vi "Dashboard Main.vi"() -> ()   [LabVIEW 2017]
uses:
  <vilib>/Utility/miscctls.llb/LVRowAndColumnTypeDef.ctl
  <vilib>/event_ctls.llb/eventvkey.ctl
  <vilib>/Rock Robotics/Network Tables/NT Read Numeric Array.vi
  <vilib>/Rock Robotics/Network Tables/NT Read Boolean Array.vi
  <vilib>/Rock Robotics/Network Tables/NT Write Boolean Array.vi
  <vilib>/Utility/file.llb/Read Delimited Spreadsheet (DBL).vi
  <vilib>/Rock Robotics/Network Tables/NT Write Numeric Array.vi
  <vilib>/Utility/file.llb/Write Delimited Spreadsheet (DBL).vi
  <vilib>/Rock Robotics/WPI/Dashboard/WPI_DashboardLogging Global.vi
panel:
  in  "Camera Settings Right":T1={"Frame Rate"=30, "Compression"=30, "Size"=1, "DB Camera Config"=FALSE} {"Frame Rate" scale=1.0..30.0; "Compression" scale=100.0..-1.0; "Size" items=["640x480", "320x240", "160x120"]}
  in  "Camera Name Right":string(combo)="No Camera Selection"
  out "Camera Info":cluster{"Mbps LED":bool, "Mbps":dbl, "fps":dbl} {"fps" format="%#.1g"; "Mbps" format="%#.1g"}
  in  "Camera Settings":T1={"Frame Rate"=30, "Compression"=30, "Size"=1, "DB Camera Config"=FALSE} {"Frame Rate" scale=1.0..30.0; "Compression" scale=100.0..-1.0; "Size" items=["640x480", "320x240", "160x120"]}
  in  "TCP":refnum<k5>
  in  "Rec Mode":enum32{"Stop", "Record", "Playback"}(radio)
  out "Robot IP":string
  out "Image Message":string="Timeout in Camera Communications"
  in  "Dashboard Tab":T2(tab)
  out "NT Connection":bool
  out "MotorChart R":cluster{"Numeric":dbl, "Numeric":dbl}(graph)
  out "MotorChart L":cluster{"Numeric":dbl, "Numeric":dbl}(graph)
  out "MotorSliders R":cluster{"MotorSlide1":dbl, "MotorSlide2":dbl} {"MotorSlide2" scale=-1.0..1.0 scale format="%#_2e"; "MotorSlide1" scale=-1.0..1.0 scale format="%#_2e"}
  out "MotorSliders L":cluster{"MotorSlide1":dbl, "MotorSlide2":dbl} {"MotorSlide2" scale=-1.0..1.0 scale format="%#_2e"; "MotorSlide1" scale=-1.0..1.0 scale format="%#_2e"}
  out "JS1 Z":dbl(slide) scale=-1.0..1.0 scale format="%#_2e"
  out "JS1 Graph":cluster{"X":dbl, "Y":dbl}[](graph)
  out "JS1 Buttons":T3
  out "JS2 Z":dbl(slide) scale=-1.0..1.0 scale format="%#_2e"
  out "JS2 Graph":cluster{"X":dbl, "Y":dbl}[](graph)
  out "JS2 Buttons":T3
  out "Mode":T4(ring)=enum."Auto Disabled"
  out "Gear State":string="Waiting...."
  out "Ramps":bool[](array[boolean])
  out "Camera Image Right":T5(plugin-control)
  in  "DB/String 9":string
  in  "DB/String 8":string
  in  "DB/String 7":string
  in  "DB/String 6":string
  in  "DB/String 5":string
  in  "DB/String 4":string
  in  "DB/String 3":string
  in  "DB/String 2":string
  in  "DB/String 1":string
  in  "DB/String 0":string
  in  "DB/Slider 0":dbl(slide) scale=0.0..5.0
  in  "DB/Slider 1":dbl(slide) scale=0.0..5.0
  in  "DB/Slider 2":dbl(slide) scale=0.0..5.0
  in  "DB/Slider 3":dbl(slide) scale=0.0..5.0
  out "DB/LED 3":bool
  out "DB/LED 2":bool
  out "DB/LED 1":bool
  out "DB/LED 0":bool
  in  "DB/Button 3":bool
  in  "DB/Button 2":bool
  in  "DB/Button 1":bool
  in  "DB/Button 0":bool caption="New Name"
  in  "Test Slider":dbl(slide) scale=0.0..100.0 scale format="%#_3g"
  in  "On/Off":bool caption="Solenoid"
  in  "Test Name":u16(ring) items=["Select the test to run..."]
  in  "Test Tree":string(tree)
  in  "Motor":cluster{"Value":dbl, "Enable":bool} {"Value" scale=-1.0..1.0 scale format="%#_3g"}
  out "Progress":T6 {"Test Progress" scale=0.0..100.0}
  in  "Rev/Fwd":cluster{"Forward":bool, "Reverse":bool}
  in  "Test Ring":u16(ring) items=["Monochrome", "Color"]
  out "Cmd Status":string
  in  "Execute Command":bool
  in  "Command Params":string[][](table)
  in  "Command Selection":i32(listbox)
  in  "CheckList":i32(listbox)
  out "Tree":string(tree)
  out "new picture":picture
  in  "Starting Pos":i16(slide)=128 scale=340.0..50.0
  in  "Right String":string
  in  "Left String":string
  in  "Load Left Auto":bool
  in  "Save Left Auto":bool
  in  "Save Right Auto":bool
  in  "Load Right Auto":bool
  in  "Select Auto":string(combo)="Select Autonomous ..."
  in  "Turn":dbl[](array[slide]) scale=0.0..1.0
  out "Speed Tuning":cluster{"yi":dbl[], "ramp data":dbl[]}[](graph)
  out "Rotation Tuning":cluster{"yi":dbl[], "ramp data":dbl[]}[](graph)
  in  "Ramps":bool
  in  "Shifting":bool
  in  "STOP":bool
  in  "Save":bool
  in  "Speed":dbl[](array[slide]) scale=0.0..1.0
  in  "Load":bool
  out "Camera Image":T5(plugin-control)
  out "Background":bool
  in  "Camera Name":string(combo)="No Camera Selection"
  # "HW"
  # "HW"
  # "Joysticks"
  # "Drive Motors"
  # "Front"
  # "Right"
  # "Left"
  # "Back"
  # "This tab is a great place for autonomous settings and robot-specific values.\nPlace controls and indicators inside this tab and match name to\nDashboard Variables on robot. You can also delete this comment."
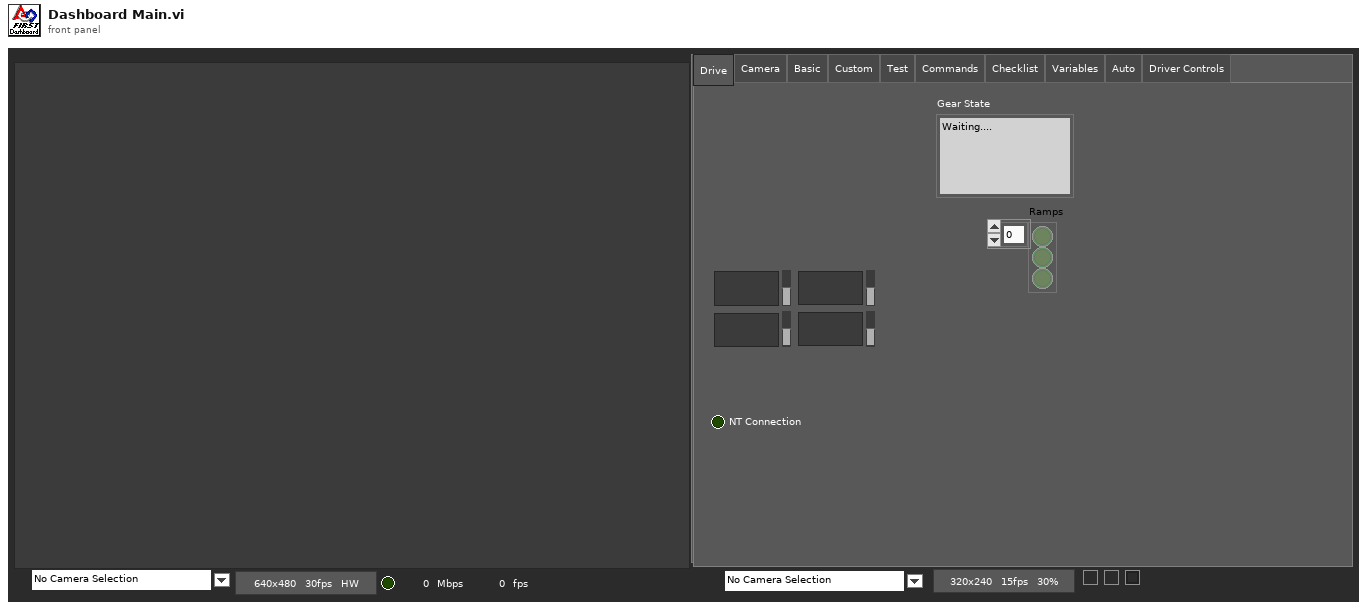
[diagram p1: front panel]
types:
  T1 = cluster{"Frame Rate":i32, "Compression":i32, "Size":u16, "DB Camera Config":bool}
  T2 = enum32{"Drive", "Camera", "Basic", "Custom", "Test", "Commands", "Checklist", "Variables", "Auto", "Driver Controls"}
  T3 = cluster{bool, bool, bool, bool, bool, bool, bool, bool, bool, bool, bool, bool}
  T4 = enum8{"Tele-Op Disabled", "Tele-Op Enabled", "Auto Disabled", "Auto Enabled", "Test Disabled", "Test Enabled", "Disconnected", "No Code", "E-Stop"}
  T5 = typedef "IMAQ Image.ctl" = refnum<image>
  T6 = cluster{"Test Progress":u8, "Test Progress Text":string}
  T7 = cluster{"Save Path":path, "Interval (s)":dbl, "Keep":i32}
  T8 = enum32{"Drive", "Camera", "Basic", "Custom", "Test", "Commands", "Checklist", "Variables"}
  T9 = typedef "Image Type" = u32
  T10 = cluster{"IDs":cluster{"RPC field ID":u16, "Unique ID":u16}, "String":string}
  T11 = cluster{"Error Strings":string, "Disable Counts":cluster{u16, u16}, "Rail Faults":cluster{u16, u16, u16}, "Robot IP":string, "DB Mode":u8, "Event Info":cluster{"Name":string, "Type":u8, "Number":u16, "Replay":u8}}
  T12 = cluster{"Storage":cluster{"Disk Free":u64, "RAM Block":u32, "RAM free":u32}, "CPU Utilization":cluster{"CPU % ISR":sgl, "CPU % Time Crit":sgl, "CPU % Timed Str":sgl, "CPU % High":sgl, "CPU % Above":sgl, "CPU % Normal":sgl, "CPU % Low":sgl}, "CAN":cluster{"% Bus Utilization":sgl, "Bus Off Cnt":u32, "TX_FIFO Full Cnt":u32, "Receive Error Cnt":u8, "Transmit Error Cnt":u8}, "HID":cluster{"HID Outputs":u32, "Rumble Low":u16, "Rumble High":u16}[]}
  T13 = cluster{"Status bits":cluster{"Test Mode":bool, "Autonomous":bool, "Enabled":bool, "Code Start":bool, "Brownout":bool, "Reserved 2":bool, "Reserved 3":bool, "E-Stop":bool}, "Code Trace":cluster{"Disabled":bool, "TeleOp":bool, "Auto":bool, "Test":bool}, "Controller Type":enum16{"unknown", "cRIO", "roboRio"}, "Code?":enum16{"unknown", "noCode", "code"}, "Battery V":dbl}
  T14 = cluster{"Control Bits":cluster{"TestMode":bool, "Autonomous":bool, "Enabled":bool, "FMS Present":bool, bool, bool, bool, "E-Stop":bool}, "Team Station ":u8, "Countdown":sgl, "Joystick Values":cluster{"Axes":dbl[], "Buttons":bool[], "POVs":i16[]}[]}
  T15 = cluster{"Axes":dbl[], "Buttons":bool[], "POVs":i16[]}[]
  T16 = cluster{"Axes":dbl[], "Buttons":bool[], "POVs":i16[]}
  T17 = cluster{"Buttons[0]":bool, "Buttons[1]":bool, "Buttons[2]":bool, "Buttons[3]":bool, "Buttons[4]":bool, "Buttons[5]":bool, "Buttons[6]":bool, "Buttons[7]":bool, "Buttons[8]":bool, "Buttons[9]":bool, "Buttons[10]":bool, "Buttons[11]":bool}
  T18 = typedef "LVBoundsTypeDef.ctl" = cluster{"Width":u32, "Height":u32}
  T19 = cluster{"Camera Image":refnum<vi>, "Dashboard Tab":refnum<vi>, "Background":refnum<vi>, "Rec Mode":refnum<vi>, "Test Slider":refnum<vi>, "On/Off ":refnum<vi>, "Test Ring":refnum<vi>, "Rev/Fwd":refnum<vi>, "Test Name":refnum<vi>, "Motor":refnum<vi>, "Progress":refnum<vi>, "CheckList":refnum<vi>, "Tree":refnum<vi>, "Test Tree":refnum<vi>, "Command Params":refnum<vi>, "Command Selection":refnum<vi>, "Execute Command":refnum<vi>, "Cmd Status":refnum<vi>, "Camera Settings":refnum<vi>, "Camera Name":refnum<vi>, "Camera Info":refnum<vi>, "Camera Settings Right":refnum<vi>, "Camera Name Right":refnum<vi>, "Camera Image Right":refnum<vi>}
  T20 = cluster{"Camera Name":string, string, "Saved DB Images Info":cluster{"Save Path":path, "Interval (s)":dbl, "Keep":i32}}
  T21 = cluster{"Camera Name Right":string, string, "Saved DB Images Info":cluster{"Save Path":path, "Interval (s)":dbl, "Keep":i32}}
  T22 = cluster{"Operation":enum16{"Update", "Clear"}, "Color Box":u32}[]
  T23 = typedef "eventvkey.ctl" = enum16{"ASCII", "Enter", "Return", "Shift", "Ctrl", "Alt", "Cmd", "Opt", "Caps", "NumLock", "Clear", "Break", "Up", "Down", "Left", "Right", "Insert", "Delete", "Home", "End", "PageUp", "PageDown", "Escape", "Help", "Pause", "ScrollLock", "F1", "F2", "F3", "F4", "F5", "F6", "F7", "F8", "F9", "F10", "F11", "F12", "F13", "F14", "F15", "F16", "F17", "F18", "F19", "F20", "F21", "F22", "F23", "F24", "Play", "VolumeUp", "VolumeDown", "Mute", "Two Byte Char"}
  T24 = cluster{"Image Size":bool, "Image Type":bool, "Pixel Value":bool, "ROI Information":bool, "Zoom Factor":bool}
  T25 = cluster{"Operation":enum16{"Update", "Clear"}, "Color Box":u32}
  T26 = typedef "LVRowAndColumnTypeDef.ctl" = cluster{"Row":i32, "Column":i32}
  T27 = cluster{"Shift":bool, "Ctrl":bool, "Alt":bool, "Cmd":bool, "Opt":bool}
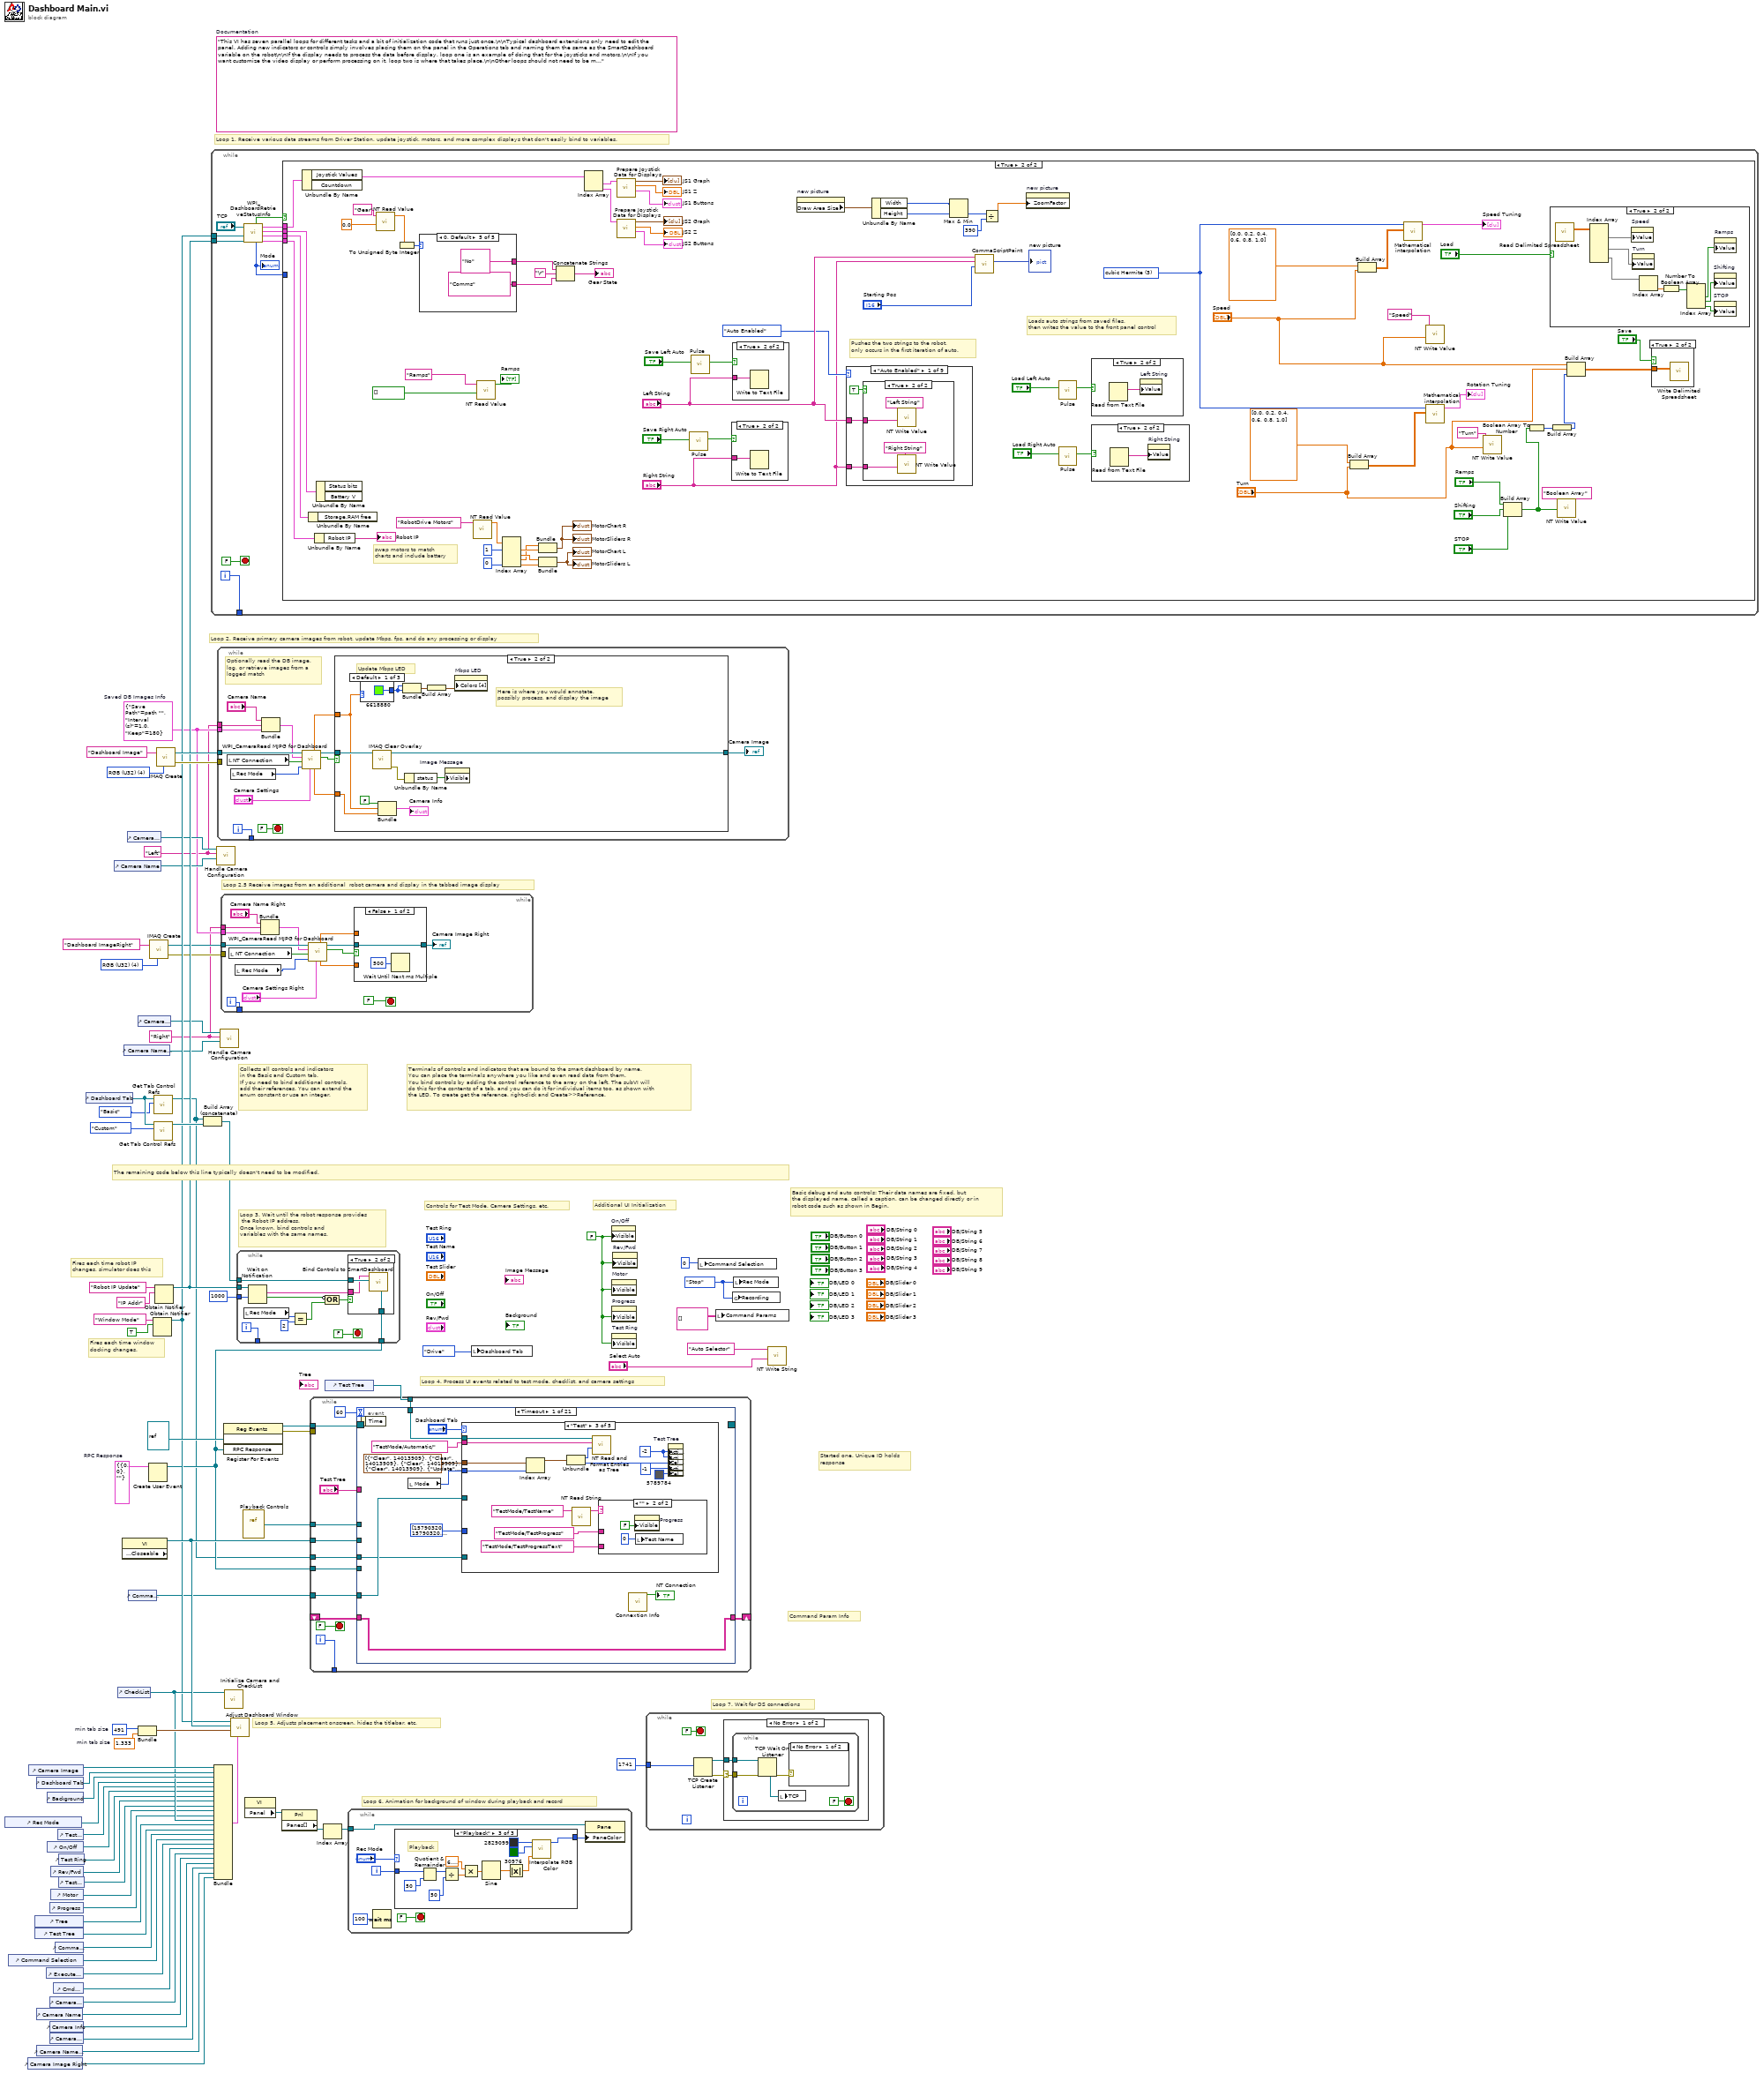
[diagram p0: block diagram]
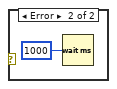
[diagram p3: hidden frame]
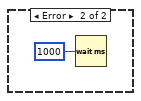
[diagram p4: hidden frame]
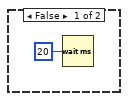
[diagram p5: hidden frame]
diagram:
  w3 = T7 {"Save Path"=path "", "Interval (s)"=1.0, "Keep"=180}  # Saved DB Images Info
  w2 = "Right"
  w1 = "Left"
  w13 = T9 4 items=["Grayscale (U8)", "Grayscale (I16)", "Grayscale (SGL)", "Complex (CSG)", "RGB (U32)", "HSL (U32)", "RGB (U64)"] ("Image Type")
  w29 = T10 {"IDs"={"RPC field ID"=0, "Unique ID"=0}, "String"=""}  # RPC Response
  w52 = 491  # min tab size
  w51 = 1.333  # min tab size
  w59 = enum32{"Stop", "Record", "Playback"}."Stop" ("Rec Mode")
  w36 = FALSE ("Visible")
  (unwired) "This VI has seven parallel loops for different tasks and a bit of initialization code that runs just once.\n\nTypical dashboard extensions only need to edit the panel. Adding new indicators or controls simply involves placing them on the panel in the Operations tab and naming them the same as the SmartDashboard variable on the robot\n\nIf the display needs to process the data before display, loop one is an example of doing that for the joysticks and motors.\n\nIf you want customize the video display or perform processing on it, loop two is where that takes place.\n\nOther loops should not need to be modified. They are pretty standard, and document the task they perform."  # Documentation
  w76 = T9 4 items=["Grayscale (U8)", "Grayscale (I16)", "Grayscale (SGL)", "Complex (CSG)", "RGB (U32)", "HSL (U32)", "RGB (U64)"] ("Image Type")
  # "Loop 2.5 Receive images from an additional  robot camera and display in the tabbed image display"
  # "Command Param Info"
  # "Started one, Unique ID holds\nresponse"
  # "Loop 7. Wait for DS connections"
  # "Basic debug and auto controls: Their data names are fixed, but\nthe displayed name, called a caption, can be changed directly or in\nrobot code such as shown in Begin."
  # "Controls for Test Mode, Camera Settings, etc."
  # "Additional UI Initialization"
  # "Loop 6. Animation for background of window during playback and record"
  # "Fires each time robot IP\nchanges, simulator does this"
  # "Fires each time window\ndocking changes."
  # "Collects all controls and indicators\nin the Basic and Custom tab.\nIf you need to bind additional controls,\nadd their references. You can extend the\nenum constant or use an integer."
  # "The remaining code below this line typically doesn't need to be modified."
  # "Loop 4. Process UI events related to test mode, checklist, and camera settings"
  # "Terminals of controls and indicators that are bound to the smart dashboard by name.\nYou can place the terminals anywhere you like and even read data from them.\nYou bind controls by adding the control reference to the array on the left. The subVI will\ndo this for the contents of a tab, and you can do it for individual items too, as shown with\nthe LED. To create get the reference, right-click and Create>>Reference."
  # "Loop 3. Wait until the robot response provides\n the Robot IP address.\nOnce known, bind controls and\nvariables with the same names."
  # "Loop 5. Adjusts placement onscreen, hides the titlebar, etc."
  # "Loop 1. Receive various data streams from Driver Station, update joystick, motors, and more complex displays that don't easily bind to variables."
  # "Loop 2. Receive primary camera images from robot, update Mbps, fps, and do any processing or display"
  n1 = control-ref of="Rec Mode"() -> (w42:refnum<vi>)
  n2 = control-ref of="Command Selection"() -> (w28:refnum<vi>)
  n3 = control-ref of="Camera Image Right"() -> (w6:refnum<vi>)
  n4 = control-ref of="Camera Image"() -> (w54:refnum<vi>)
  n5 = control-ref of="Tree"() -> (w46:refnum<vi>)
  n6 = control-ref of="Test Tree"() -> (w45:refnum<vi>)
  n7 = control-ref of="Dashboard Tab"() -> (w53:refnum<vi>)
  n8 = control-ref of="Camera Name"() -> (w19:refnum<vi>)
  n9 = control-ref of="Camera Name Right"() -> (w7:refnum<vi>)
  n10 = control-ref of="Execute Command"() -> (w30:refnum<vi>)
  n11 = control-ref of="Background"() -> (w49:refnum<vi>)
  n12 = control-ref of="On/Off"() -> (w40:refnum<vi>)
  n13 = control-ref of="Progress"() -> (w37:refnum<vi>)
  n14 = control-ref of="Camera Settings"() -> (w20:refnum<vi>)
  n15 = control-ref of="Camera Info"() -> (w18:refnum<vi>)
  n16 = control-ref of="Camera Settings Right"() -> (w8:refnum<vi>)
  n17 = control-ref of="Rev/Fwd"() -> (w38:refnum<vi>)
  n18 = control-ref of="Motor"() -> (w43:refnum<vi>)
  n19 = control-ref of="Cmd Status"() -> (w24:refnum<vi>)
  n20 = control-ref of="Command Params"() -> (w31:refnum<vi>)
  n21 = control-ref of="Test Slider"() -> (w41:refnum<vi>)
  n22 = control-ref of="Test Ring"() -> (w39:refnum<vi>)
  n23 = control-ref of="Test Name"() -> (w44:refnum<vi>)
  n24 = control-ref of="Dashboard Tab"() -> (w57:refnum<vi>)
  n25 = control-ref of="Camera Name"() -> (w21:refnum<vi>)
  n26 = control-ref of="CheckList"() -> (w47:refnum<vi>)
  n27 = property class="VI" props=["Front Panel.Closeable"]() -> (reference out=w58:refnum<vi>)  [unwired: 2 in, 2 out]
  n28 = control-ref of="Camera Name Right"() -> (w9:refnum<vi>)
  n29 = control-ref of="Camera Settings"() -> (w22:refnum<vi>)
  n30 = control-ref of="Command Params"() -> (w23:refnum<vi>)
  n31 = control-ref of="Camera Settings Right"() -> (w10:refnum<vi>)
  n32 = Bundle("min tab size"=w52, "min tab size"=w51) -> (w50:cluster{"min tab size":i32, "min tab size":dbl})  [unwired: 1 in]
  n33 = Create User Event(user event datatype=w29) -> (user event=w25:refnum<user-event>)  [unwired: 1 in, 1 out]
  n34 = call "IMAQ Create"("Image Name"="Dashboard ImageRight", "Image Type"=w13) -> ("New Image"=w12:T5, "error out"=w11:errorcluster)  [unwired: 2 in, 1 out]
  n35 = Obtain Notifier(name (unnamed)="Window Mode", notification data type=TRUE) -> (notifier out=w34:refnum<notifier>)  [unwired: 2 in, 2 out]
  n36 = call <vilib>:"Get Tab Control Refs.vi"("Page Index"=T8."Basic" ("Dashboard Tab"), "TabControl in"=w57) -> ("ControlsOnPage"=w17:refnum<vi>[])  [unwired: 9 in]
  n37 = call <vilib>:"Get Tab Control Refs.vi"("Page Index"=T8."Custom" ("Dashboard Tab"), "TabControl in"=w57) -> ("ControlsOnPage"=w56:refnum<vi>[])  [unwired: 9 in]
  n38 = Obtain Notifier(name (unnamed)="Robot IP Update", notification data type="IP Addr" ("name (unnamed)")) -> (notifier out=w35:refnum<notifier>)  [unwired: 2 in, 2 out]
  n39 = call "IMAQ Create"("Image Name"="Dashboard Image", "Image Type"=w76) -> ("New Image"=w74:T5, "error out"=w73:errorcluster)  [unwired: 2 in, 1 out]
  n40 = Build Array (concatenate)(w17, w56) -> (w55:refnum<vi>[])
  n41 = while {
    tunnel: [w86] -> _
    tunnel: w35 -> [w80]
    tunnel: w34 -> [w77]
    i -> [w86]
    stop <- FALSE stop-if-true
    n42 = call <vilib>:"WPI_DashboardRetrieveStatusInfo.vi"("Binding Refnum"=w80, "Window Mode Notifier"=w77, "TCP Cnx"="TCP") -> ("Power and Errors"=w81:T11, "Robot Metrics"=w84:T12, "Status Info"=w85:T13, "Control Info"=w82:T14, "Robot Mode"=w79:T4, "Process?"=w83:bool)  [unwired: 3 in]
    "Mode" <- w79
    n43 = case shown="True" w83 {
      tunnel: w85 -> [_ w163]
      tunnel: w84 -> [_ w162]
      tunnel: w82 -> [_ w161]
      tunnel: w81 -> [_ w160]
      tunnel: w79 -> [_ _]
      frame False {
        n44 = Wait (ms)(milliseconds to wait=u32 20) -> ()  [unwired: 1 out]
      }
      frame True {
        w109 = 3 items=["nearest", "linear", "spline", "cubic Hermite", "Lagrange"] ("Method")
        # "Pushes the two strings to the robot,\nonly occurs in the first iteration of auto."
        # "Loads auto strings from saved files,\nthen writes the value to the front panel control"
        # "swap motors to match\ncharts and include battery"
        n45 = Unbundle By Name(w161) -> ("Joystick Values"=w151:T15)  [unwired: 1 out]
        n46 = Unbundle By Name(w162) -> ()  [unwired: 1 out]
        n47 = Unbundle By Name(w160) -> ("Robot IP"=→"Robot IP":string)
        n48 = Unbundle By Name(w163) -> ()  [unwired: 2 out]
        n49 = call-poly <vilib>:"NT Read Value.vi"("Default Value"=0.0, "Name"="Gear") -> ("Numeric"=w138:dbl)  [unwired: 8 in, 1 out]
        n50 = To Unsigned Byte Integer(number=w138) -> (unsigned 8bit integer=w139:u8)
        n51 = case shown="0, Default" w139 {
          tunnel: ["Low" "High" "Low" "High" "No"] -> w135
          tunnel: ["Manual" "Manual" "Automatic" "Automatic" "Comms"] -> w133
          frame 1 {
          }
          frame 2 {
          }
          frame 3 {
          }
          frame 4 {
          }
          frame 0, Default {
          }
        }
        n52 = call-poly <vilib>:"NT Read Value.vi"("Name"="RobotDrive Motors") -> ("Numeric Array"=w141:dbl[])  [unwired: 9 in, 1 out]
        n53 = call-poly <vilib>:"NT Read Value.vi"("Default Value"=bool[] [], "Name"="Ramps") -> ("Boolean Array"=→"Ramps":bool[])  [unwired: 8 in, 1 out]
        n54 = Index Array(array=w141, index #1=1, index #4=0) -> (element #1=w155:dbl, element #2=w156:dbl, element #3=w154:dbl, element #4=w159:dbl)  [unwired: 2 in]
        n55 = Bundle("Numeric"=w154, "Numeric"=w155) -> (→"MotorChart R" →"MotorSliders R":cluster{"Numeric":dbl, "Numeric":dbl})  [unwired: 1 in]
        n56 = Bundle("Numeric"=w156, "Numeric"=w159) -> (→"MotorChart L" →"MotorSliders L":cluster{"Numeric":dbl, "Numeric":dbl})  [unwired: 1 in]
        n57 = Concatenate Strings(w135, "\r", w133) -> (→"Gear State":string)
        n58 = Index Array(array=w151) -> (element #1=w150:T16, element #2=w146:T16)  [unwired: 2 in]
        n59 = call "Prepare Joystick Data for Displays.vi"("Joystick Values"=w146) -> ("Buttons"=→"JS2 Buttons":T17, "Z Axis"=→"JS2 Z":dbl, "Cartesian Data"=→"JS2 Graph":cluster{"X axis":dbl, "X axis":dbl}[])  [unwired: 8 in]
        n60 = call "Prepare Joystick Data for Displays.vi"("Joystick Values"=w150) -> ("Buttons"=→"JS1 Buttons":T17, "Z Axis"=→"JS1 Z":dbl, "Cartesian Data"=→"JS1 Graph":cluster{"X axis":dbl, "X axis":dbl}[])  [unwired: 8 in]
        n61 = call "Pulse.vi"("Input"="Save Right Auto") -> ("Output"=w126:bool)  [unwired: 10 in]
        n62 = call "Pulse.vi"("Input"="Save Left Auto") -> ("Output"=w122:bool)  [unwired: 10 in]
        n63 = case shown="True" w126 {
          tunnel: "Right String" -> [_ w181]
          frame False {
          }
          frame True {
            n64 = Write to Text File(text=w181) -> ()  [unwired: 3 in, 3 out]
          }
        }
        n65 = case shown="True" w122 {
          tunnel: "Left String" -> [_ w184]
          frame False {
          }
          frame True {
            n66 = Write to Text File(text=w184) -> ()  [unwired: 3 in, 3 out]
          }
        }
        n67 = property on="new picture" class="Pict"() -> ("Draw Area Size"=w114:T18)  [unwired: 2 in, 2 out]
        n68 = case shown="\"Auto Enabled\"" T4."Auto Enabled" ("Robot Mode") {
          tunnel: "Left String" -> [w176 _ _ _ _ _ _ _ _]
          tunnel: "Right String" -> [w175 _ _ _ _ _ _ _ _]
          frame "Auto Enabled" {
            n69 = case shown="True" TRUE {
              tunnel: w176 -> [_ w180]
              tunnel: w175 -> [_ w179]
              frame False {
              }
              frame True {
                n70 = call-poly <vilib>:"NT Write Value.vi"("String"=w180, "Name"="Left String") -> ()  [unwired: 9 in, 1 out]
                n71 = call-poly <vilib>:"NT Write Value.vi"("String"=w179, "Name"="Right String") -> ()  [unwired: 9 in, 1 out]
              }
            }
          }
          frame "Test Disabled" {
          }
          frame "Test Enabled" {
          }
          frame "Disconnected" {
          }
          frame "No Code" {
          }
          frame "E-Stop" {
          }
          frame "Auto Disabled" {
          }
          frame "Tele-Op Enabled" {
          }
          frame "Tele-Op Disabled" {
          }
        }
        n72 = Unbundle By Name(w114) -> ("Width"=w118:u32, "Height"=w117:u32)
        n73 = Max & Min(x=w118, y=w117) -> (min(x,y)=w116:u32)  [unwired: 1 out]
        n74 = call "CommaScriptPaint.vi"("Starting Pos"="Starting Pos", "string 2"="Right String", "string"="Left String") -> ("new picture"=→"new picture":picture)  [unwired: 7 in, 1 out]
        n75 = Divide(x=w116, y=u32 390) -> (x/y=w113:dbl)
        n76 = property on="new picture" class="Pict"("ZoomFactor"=w113) -> ()  [unwired: 2 in, 2 out]
        n77 = call "Pulse.vi"("Input"="Load Left Auto") -> ("Output"=w123:bool)  [unwired: 10 in]
        n78 = call "Pulse.vi"("Input"="Load Right Auto") -> ("Output"=w129:bool)  [unwired: 10 in]
        n79 = case shown="True" w123 {
          frame False {
          }
          frame True {
            n80 = Read from Text File() -> (text=w183:string)  [unwired: 4 in, 3 out]
            n81 = property on="Left String" class="Str"("Value"=w183) -> ()  [unwired: 2 in, 2 out]
          }
        }
        n82 = case shown="True" w129 {
          frame False {
          }
          frame True {
            n83 = Read from Text File() -> (text=w182:string)  [unwired: 4 in, 3 out]
            n84 = property on="Right String" class="Str"("Value"=w182) -> ()  [unwired: 2 in, 2 out]
          }
        }
        n85 = Build Array(dbl[] [0.0, 0.2, 0.4, 0.6, 0.8, 1.0] ("Speed 2"), "Turn") -> (w91:dbl[][])
        n86 = Build Array(dbl[] [0.0, 0.2, 0.4, 0.6, 0.8, 1.0] ("Speed 2"), "Speed") -> (w100:dbl[][])
        n87 = call "Mathematical interpolation.vi"("Input data"=w100, "Method"=w109) -> ("1D Interpolation Graph"=→"Speed Tuning":cluster{"yi":dbl[], "ramp data":dbl[]}[])  [unwired: 8 in, 1 out]
        n88 = call-poly <vilib>:"NT Write Value.vi"("Numeric Array"="Speed", "Name"="Speed") -> ()  [unwired: 9 in, 1 out]
        n89 = call "Mathematical interpolation.vi"("Input data"=w91, "Method"=w109) -> ("1D Interpolation Graph"=→"Rotation Tuning":cluster{"yi":dbl[], "ramp data":dbl[]}[])  [unwired: 8 in, 1 out]
        n90 = call-poly <vilib>:"NT Write Value.vi"("Numeric Array"="Turn", "Name"="Turn") -> ()  [unwired: 9 in, 1 out]
        n91 = Build Array("Ramps", "Shifting", "STOP") -> (w99:bool[])
        n92 = Boolean Array To Number(Boolean array=w99) -> (number=w98:u32)
        n93 = case shown="True" "Load" {
          frame False {
          }
          frame True {
            n94 = call-poly <vilib>:"Read Delimited Spreadsheet.vi"() -> ("all rows"=w172:dbl[][])  [unwired: 10 in, 5 out]
            n95 = Index Array(array=w172) -> (element #1=w171:dbl[], element #2=w170:dbl[], element #3=w169:dbl[])  [unwired: 6 in]
            n96 = property on="Speed" class="Arr (strict)"("Value"=w171) -> ()  [unwired: 2 in, 2 out]
            n97 = property on="Turn" class="Arr (strict)"("Value"=w170) -> ()  [unwired: 2 in, 2 out]
            n98 = Index Array(array=w169) -> (element=w168:dbl)  [unwired: 1 in]
            n99 = Number To Boolean Array(number=w168) -> (Boolean array=w167:bool[])
            n100 = Index Array(array=w167) -> (element #1=w166:bool, element #2=w165:bool, element #3=w164:bool)  [unwired: 3 in]
            n101 = property on="Shifting" class="Bool (strict)"("Value"=w165) -> ()  [unwired: 2 in, 2 out]
            n102 = property on="STOP" class="Bool (strict)"("Value"=w164) -> ()  [unwired: 2 in, 2 out]
            n103 = property on="Ramps" class="Bool (strict)"("Value"=w166) -> ()  [unwired: 2 in, 2 out]
          }
        }
        n104 = Build Array(w98) -> (w97:u32[])
        n105 = call-poly <vilib>:"NT Write Value.vi"("Boolean Array"=w99, "Name"="Boolean Array") -> ()  [unwired: 9 in, 1 out]
        n106 = Build Array("Speed", "Turn", w97) -> (w96:dbl[][])
        n107 = case shown="True" "Save" {
          tunnel: w96 -> [_ w173]
          frame False {
          }
          frame True {
            n108 = call-poly <vilib>:"Write Delimited Spreadsheet.vi"("2D data"=w173) -> ()  [unwired: 13 in, 2 out]
          }
        }
      }
    }
  }
  n109 = Bundle("Camera Image"=w54, "Dashboard Tab"=w53, "Background"=w49, "Rec Mode"=w42, "Test Slider"=w41, "On/Off"=w40, "Test Ring"=w39, "Rev/Fwd"=w38, "Test Name"=w44, "Motor"=w43, "Progress"=w37, "CheckList"=w47, "Tree"=w46, "Test Tree"=w45, "Command Params"=w31, "Command Selection"=w28, "Execute Command"=w30, "Cmd Status"=w24, "Camera Settings"=w20, "Camera Name"=w19, "Camera Info"=w18, "Camera Settings Right"=w8, "Camera Name Right"=w7, "Camera Image Right"=w6) -> (w48:T19)  [unwired: 1 in]
  n110 = call "Handle Camera Configuration.vi"("CameraNameRef"=w21, "Display Name"=w1, "ClusterRef"=w22) -> ()  [unwired: 9 in]
  n111 = while {
    tunnel: w74 -> [w207]
    tunnel: w73 -> [_]
    tunnel: [w208] -> _
    tunnel: w3 -> [w198]
    tunnel: w1 -> [w195]
    i -> [w208]
    stop <- FALSE stop-if-true
    # "Optionally read the DB image,\nlog, or retrieve images from a\nlogged match"
    n112 = local read "NT Connection"() -> (w199:bool)
    n113 = local read "Rec Mode"() -> (w203:enum32{"Stop", "Record", "Playback"})
    n114 = Bundle("Camera Name"="Camera Name", w195, "Saved DB Images Info"=w198) -> (w197:T20)  [unwired: 1 in]
    n115 = call <vilib>:"WPI_CameraRead MJPG for Dashboard.vi"("Camera Settings"="Camera Settings", "Rec Mode"=w203, "NT Connection"=w199, "Capture Info"=w197, "Refnum in"=w207) -> ("Active"=w205:bool, "Refnum out"=w206:T5, "FPS"=w204:dbl, "Bandwidth (Mbps)"=w202:dbl)  [unwired: 3 in]
    n116 = case shown="True" w205 {
      tunnel: w206 -> [w210 w221]
      tunnel: w202 -> [_ w218]
      tunnel: w204 -> [_ w219]
      tunnel: [w210 w215] -> w200
      frame False {
        w212 = u32 1985280 ("Color Box")
        # "Sleep for 500ms"
        n117 = Bundle("Color Box"=w212, "Color Box"=w212) -> (w213:cluster{"Color Box":u32, "Color Box":u32})  [unwired: 1 out]
        n118 = Build Array(w213) -> (w211:cluster{"Color Box":u32, "Color Box":u32}[])
        n119 = property on="Mbps LED" class="Bool (strict)"("Colors [4]"=w211) -> ()  [unwired: 2 in, 2 out]
        n120 = Wait Until Next ms Multiple(millisecond multiple=u32 500) -> ()  [unwired: 1 out]
      }
      frame True {
        # "Here is where you would annotate,\npossibly process, and display the image"
        # "Update Mbps LED"
        n121 = case shown="Default" w218 {
          tunnel: [u32 6618880 ("Color Box") u32 16776722 ("Color Box") u32 16716800 ("Color Box")] -> w222
          frame Default {
          }
          frame 4, 5 {
          }
          frame 6.. {
          }
        }
        n122 = call "IMAQ Clear Overlay"("Image"=w221) -> ("error out"=w224:errorcluster, "Image Out"=w215:T5)  [unwired: 2 in, 7 out]
        n123 = Bundle(FALSE, "Bandwidth (Mbps)"=w218, "FPS"=w219) -> (→"Camera Info":cluster{bool, "Bandwidth (Mbps)":dbl, "FPS":dbl})  [unwired: 1 in]
        n124 = Bundle("Color Box"=w222, "Color Box"=w222) -> (w223:cluster{"Color Box":u32, "Color Box":u32})  [unwired: 1 out]
        n125 = Unbundle By Name(w224) -> ("status"=w225:bool)
        n126 = Build Array(w223) -> (w220:cluster{"Color Box":u32, "Color Box":u32}[])
        n127 = property on="Image Message" class="Str"("Visible"=w225) -> ()  [unwired: 2 in, 2 out]
        n128 = property on="Mbps LED" class="Bool (strict)"("Colors [4]"=w220) -> ()  [unwired: 2 in, 2 out]
      }
    }
    "Camera Image" <- w200
  }
  n129 = call "Handle Camera Configuration.vi"("CameraNameRef"=w9, "Display Name"=w2, "ClusterRef"=w10) -> ()  [unwired: 9 in]
  n130 = while {
    tunnel: w12 -> [w243]
    tunnel: w11 -> [_]
    tunnel: [w238] -> _
    tunnel: w3 -> [w232]
    tunnel: w2 -> [w229]
    i -> [w238]
    stop <- FALSE stop-if-true
    n131 = local read "NT Connection"() -> (w233:bool)
    n132 = local read "Rec Mode"() -> (w242:enum32{"Stop", "Record", "Playback"})
    n133 = Bundle("Camera Name Right"="Camera Name Right", w229, "Saved DB Images Info"=w232) -> (w231:T21)  [unwired: 1 in]
    n134 = call <vilib>:"WPI_CameraRead MJPG for Dashboard.vi"("Camera Settings"="Camera Settings Right", "Rec Mode"=w242, "NT Connection"=w233, "Capture Info"=w231, "Refnum in"=w243) -> ("Active"=w237:bool, "Refnum out"=w240:T5, "FPS"=w235:dbl, "Bandwidth (Mbps)"=w236:dbl)  [unwired: 3 in]
    n135 = case shown="False" w237 {
      tunnel: w240 -> [w244 w246]
      tunnel: w236 -> [_ _]
      tunnel: w235 -> [_ _]
      tunnel: [w244 w246] -> w234
      frame False {
        n136 = Wait Until Next ms Multiple(millisecond multiple=u32 500) -> ()  [unwired: 1 out]
      }
      frame True {
      }
    }
    "Camera Image Right" <- w234
  }
  n137 = register-events(refnum<vi> refnum, w25) -> (reference out=w63:refnum<event-registration>, error out=w62:errorcluster)  [unwired: 2 in]
  n138 = call "Initialize Camera and CheckList.vi"("ListBox in"=w47) -> ()  [unwired: 11 in]
  n139 = call "Adjust Dashboard Window.vi"("Sizing Refnums"=w48, "Size Constraints"=w50, "VI"=w58, "WIn Mode"=w34) -> ()  [unwired: 8 in]
  n140 = while {
    tunnel: w55 -> [w258]
    tunnel: w35 -> [w256]
    tunnel: [w254] -> _
    tunnel: u32 1000 ("milliseconds to wait") -> [w253]
    tunnel: w25 -> [w247]
    i -> [w254]
    stop <- FALSE stop-if-true
    n141 = local read "Rec Mode"() -> (w249:enum32{"Stop", "Record", "Playback"})
    n142 = Wait on Notification(notifier=w256, timeout in ms (-1)=w253) -> (notification=w255:string, timed out?=w251:bool)  [unwired: 2 in, 2 out]
    n143 = Equal?(x=w249, y=u16 2 ("Rec Mode")) -> (x = y?=w250:bool)
    n144 = Compound Arithmetic op=OR(invert w251, w250) -> (w252:bool)
    n145 = case shown="True" w252 {
      tunnel: w258 -> [_ w261]
      tunnel: w255 -> [_ w260]
      tunnel: w247 -> [_ w259]
      frame False {
      }
      frame True {
        n146 = call <vilib>:"Bind Controls to SmartDashboard.vi"("RPC ref"=w259, "Bound Control Refs"=w261, "Server IP Address"=w260) -> ()  [unwired: 9 in]
      }
    }
  }
  n147 = vi-ref "Playback Controls.vi"() -> (w64:refnum<vi>)
  n148 = property class="VI"() -> ("Panel"=w66:refnum<vi>)  [unwired: 2 in, 2 out]
  n149 = property class="Pnl"(reference=w66) -> ("Panes[]"=w67:refnum<vi>[])  [unwired: 1 in, 2 out]
  n150 = Index Array(array=w67) -> (element=w65:refnum<vi>)  [unwired: 1 in]
  n151 = control-ref of="Test Tree"() -> (w68:refnum<vi>)
  n152 = while {
    tunnel: [w271] -> _
    tunnel: w68 -> [w270]
    tunnel: w64 -> [w269]
    tunnel: w63 -> [w268]
    tunnel: w62 -> [_]
    tunnel: w58 -> [w267]
    tunnel: w25 -> [w266]
    tunnel: w23 -> [w265]
    shift-right: [w264] -> _
    shift-left: _ -> [w263]
    tunnel: w17 -> [w262]
    i -> [w271]
    stop <- FALSE stop-if-true
    n153 = event shown="[0] Timeout" {
      selector: w268 -> [_ _ _ _ _ _ _ _ _ _ _ _ _ _ _ _ _ _ _ _ _]
      dyn-events: [_ _ _ _ _ _ _ _ _ _ _ _ _ _ _ _ w531 _ _ _ _] -> _
      timeout: u32 60 ("milliseconds to wait") -> [_ _ _ _ _ _ _ _ _ _ _ _ _ _ _ _ _ _ _ _ _]
      tunnel: w270 -> [w283 _ _ _ _ _ _ _ _ _ _ _ _ _ _ _ _ _ _ _ _]
      tunnel: "Test Tree" -> [_ _ _ _ _ _ _ _ _ _ _ w498 w506 w508 w512 w520 _ _ _ _ _]
      tunnel: w269 -> [_ _ _ _ _ _ _ _ _ _ _ _ _ _ _ _ w533 _ w551 _ _]
      tunnel: w267 -> [_ _ _ _ _ _ _ _ _ _ _ _ _ _ _ _ w529 _ _ _ _]
      tunnel: w266 -> [_ _ _ _ _ _ _ _ _ _ _ _ _ _ _ _ w527 _ _ _ _]
      tunnel: w265 -> [w278 _ _ _ _ _ w449 _ _ _ _ _ _ _ _ _ _ _ _ _ _]
      tunnel: [w277 w326 w428 w433 w442 w446 w447 w456 w466 w473 w485 w497 w504 w507 w511 w519 w526 w546 w548 w552 w565] -> w264
      tunnel: w263 -> [w277 w326 w428 w433 w442 w446 w447 _ _ w473 w485 w497 w504 w507 w511 w519 w526 w546 w548 w552 w565]
      tunnel: w262 -> [w275 _ _ _ _ _ _ _ _ _ _ _ _ _ _ _ _ _ _ _ _]
      event Timeout {
        n154 = event-data() -> ()  [unwired: 1 in, 1 out]
        n155 = local read "Mode"() -> (w280:T4)
        n156 = case shown="\"Test\"" "Dashboard Tab" {
          tunnel: w283 -> [_ _ w299 _ _]
          tunnel: "TestMode/Automatic/" ("Name Pattern") -> [_ _ w298 _ _]
          tunnel: T22 [{"Operation"=enum."Clear", "Color Box"=14013909}, {"Operation"=enum."Clear", "Color Box"=14013909}, {"Operation"=enum."Clear", "Color Box"=14013909}, {"Operation"=enum."Clear", "Color Box"=14013909}, {"Operation"=enum."Update", "Color Box"=14013909}, {"Operation"=enum."Update", "Color Box"=16777215}, {"Operation"=enum."Clear", "Color Box"=14013909}, {"Operation"=enum."Clear", "Color Box"=14013909}, {"Operation"=enum."Clear", "Color Box"=14013909}] -> [_ _ w291 _ w319]
          tunnel: w280 -> [_ _ w290 _ w318]
          tunnel: u32[] [15790320, 15790320, 15790320, 15790320, 16777215, 16777215, 15790320, 15790320, 15790320] -> [_ _ _ _ w324]
          tunnel: w278 -> [_ _ _ _ w312]
          tunnel: w275 -> [_ w285 _ _ _]
          frame "Custom", Default {
          }
          frame "Basic" {
            n157 = call <vilib>:"WPI_DashboardUpdateNames.vi"("Controls on Tab"=w285) -> ()  [unwired: 11 in]
          }
          frame "Test" {
            w297 = -2 ("Active Item:Row Number")
            n158 = Index Array(array=w291, index=w290) -> (element=w292:T25)
            n159 = Unbundle(w292) -> ("Operation"=w293:enum16{"Update", "Clear"}, "Color Box"=w294:u32)
            n160 = call <vilib>:"NT Read String.vi"("Name"="TestMode/TestName") -> ("String"=w288:string)  [unwired: 9 in, 1 out]
            n161 = call <vilib>:"NT Read and Format Entries as Tree.vi"("Operation"=w293, "Name Pattern"=w298, "Tree Refnum"=w299) -> ()  [unwired: 7 in, 2 out]
            n162 = case shown="\"\"" w288 {
              tunnel: "TestMode/TestProgress" ("Name") -> [w301 _]
              tunnel: "TestMode/TestProgressText" ("Name") -> [w300 _]
              frame Default {
                n163 = call <vilib>:"NT Read Number.vi"("Name"=w301) -> ("Numeric"=w302:dbl)  [unwired: 9 in, 1 out]
                n164 = call <vilib>:"NT Read String.vi"("Name"=w300) -> ("String"=w303:string)  [unwired: 9 in, 1 out]
                n165 = Bundle("Numeric"=w302, "String"=w303) -> (→"Progress":cluster{"Numeric":dbl, "String":string})  [unwired: 1 in]
              }
              frame "" {
                n166 = property on="Progress" class="Clust (strict)"("Visible"=FALSE) -> ()  [unwired: 2 in, 2 out]
                n167 = local write "Test Name"(u16 0) -> ()
              }
            }
            n168 = property on="Test Tree" class="Tree (strict)"("Active Item Row Number"=w297, "ActiveColNum"=w297, "CellBG"=w294, "Active Item Row Number"=-1 ("Active Item:Row Number"), "CellBG"=u32 5789784 ("Color Box")) -> ()  [unwired: 2 in, 2 out]
          }
          frame "Variables" {
            w309 = string[] ["CameraPublisher", "Usage", "DB"]  # Items to initially close
            n169 = First Call?() -> (First Call?: T/F=w310:bool)
            n170 = control-ref of="Tree"() -> (w311:refnum<vi>)
            n171 = Select(t=w309, s=w310, f=string[] []) -> (s? t:f=w307:string[])
            n172 = call <vilib>:"NT Read and Format Entries as Tree.vi"("Tags to  Close"=w307, "Tree Refnum"=w311) -> ()  [unwired: 8 in, 2 out]
          }
          frame "Commands" {
            w320 = u32 5789784 ("Color Box")
            w321 = T26 {"Row"=-1, "Column"=-2} ("Active Cell:Active Cell")
            w323 = T26 {"Row"=-2, "Column"=-2} ("Active Cell:Active Cell")
            n173 = Index Array(array=w324, index=w318) -> (element=w322:u32)
            n174 = Index Array(array=w319, index=w318) -> (element=w317:T25)
            n175 = Unbundle(w317) -> ("Operation"=w316:enum16{"Update", "Clear"})  [unwired: 1 out]
            n176 = local read "Command Selection"() -> (w315:i32)
            n177 = property on="Command Selection" class="MCListbox (strict)"("ActiveCell"=w323, "CellBG"=w322, "ActiveCell"=w321, "CellBG"=w320) -> ()  [unwired: 2 in, 2 out]
            n178 = call <vilib>:"WPI_DashboardUpdate RPC Info.vi"("Operation"=w316) -> ("update"=w314:bool, "commands"=w313:string[][])  [unwired: 9 in]
            n179 = property on="Command Selection" class="MCListbox (strict)"("ItemNames"=w313) -> ()  [unwired: 2 in, 2 out]
            n180 = property on="Command Params" class="Tbl (strict)"("Active Cell"=w323, "Cell BG Color"=w322, "Active Cell"=w321, "Cell BG Color"=w320) -> ()  [unwired: 2 in, 2 out]
            n181 = call <vilib>:"WPI_DashboardUpdate Command Params.vi"("Update"=w314, "NewVal"=w315, "Commands"=w313, "Param Tbl"=w312) -> ()  [unwired: 7 in, 1 out]
          }
        }
        n182 = call <vilib>:"Connextion Info.vi"() -> ("Connected"=→"NT Connection":bool)  [unwired: 10 in, 1 out]
      }
      event "Test Tree": Value Change {
        # "Show appropriate\ncontrols"
        n183 = event-data() -> ("CtlRef"=w329:refnum<vi>, "NewVal"=w327:string)  [unwired: 1 in]
        n184 = call <vilib>:"WPI_UtilitiesGetTreeIOName.vi"("NewVal"=w327, "TreeControl in"=w329) -> ("I/O Name"=w330:string)  [unwired: 9 in]
        n185 = case shown="\"Camera\"" w330 {
          selector: w330 -> [_ w337 _ w359 w368 _]
          tunnel: w327 -> [_ _ w356 w358 _ w375]
          tunnel: cluster{string[]}[] [{["640x480", "320x240", "160x120"]}, {["Auto", "Fixed indoor", "Fixed outdoor 1", "Fixed outdoor 2", "Fixed fluorescent 1", "Fixed fluorescent 2", "Hold current"]}, {["Auto", "Flicker-free 50 Hz", "Flicker-free 60 Hz", "Hold current"]}, {["None", "Prioritize frame rate", "Prioritize image quality"]}, {["Monochrome", "Color"]}] -> [_ _ _ _ _ w374]
          frame Default {
            w332 = FALSE ("Visible")
            w331 = FALSE ("Visible")
            n186 = property on="Motor" class="Clust (strict)"("Visible"=w331) -> ()  [unwired: 2 in, 2 out]
            n187 = property on="Test Ring" class="Ring (strict)"("Visible"=w331) -> ()  [unwired: 2 in, 2 out]
            n188 = property on="Rev/Fwd" class="Clust (strict)"("Visible"=w332) -> ()  [unwired: 2 in, 2 out]
            n189 = property on="On/Off" class="Bool (strict)"("Visible"=w332) -> ()  [unwired: 2 in, 2 out]
            n190 = property on="Test Slider" class="Slide (strict)"("Visible"=w332) -> ()  [unwired: 2 in, 2 out]
          }
          frame "Analog Out", "Motor", "PWM" {
            w338 = FALSE ("Visible")
            n191 = case shown="\"Analog Out\"" w337 {
              tunnel: [1.0 ("Value") -1.0 ("Value") 0.0 ("Value")] -> w336
              tunnel: [255.0 ("Value") 1.0 ("Value") 5.0 ("Value")] -> w335
              tunnel: [128.0 ("Value") 0.0 ("Value") 0.0 ("Value")] -> w334
              tunnel: [64.0 ("Value") 0.5 ("Value") 1.0 ("Value")] -> w333
              frame "PWM" {
              }
              frame "Motor", Default {
              }
              frame "Analog Out" {
              }
            }
            n192 = property on="Motor" class="Clust (strict)"("Visible"=TRUE) -> ()  [unwired: 2 in, 2 out]
            n193 = property on="Value" class="Slide (strict)"("Value"=w334, "Scale.Minimum"=w336, "Scale.Maximum"=w335, "Scale.Increment"=w333) -> ()  [unwired: 2 in, 2 out]
            n194 = property on="On/Off" class="Bool (strict)"("Visible"=w338) -> ()  [unwired: 2 in, 2 out]
            n195 = property on="Test Slider" class="Slide (strict)"("Visible"=w338) -> ()  [unwired: 2 in, 2 out]
            n196 = property on="Test Ring" class="Ring (strict)"("Visible"=w338) -> ()  [unwired: 2 in, 2 out]
            n197 = property on="Rev/Fwd" class="Clust (strict)"("Visible"=w338) -> ()  [unwired: 2 in, 2 out]
          }
          frame "Servo" {
            w354 = FALSE ("Visible")
            n198 = call <vilib>:"NT Read Number.vi"("Name"=w356) -> ("Numeric"=w355:dbl)  [unwired: 9 in, 1 out]
            n199 = property on="Test Slider" class="Slide (strict)"("Visible"=TRUE, "Scale.Maximum"=170.0 ("Scale.Range:Maximum")) -> ()  [unwired: 2 in, 2 out]
            n200 = local write "Test Slider"(w355) -> ()
            n201 = property on="Motor" class="Clust (strict)"("Visible"=w354) -> ()  [unwired: 2 in, 2 out]
            n202 = property on="Rev/Fwd" class="Clust (strict)"("Visible"=w354) -> ()  [unwired: 2 in, 2 out]
            n203 = property on="On/Off" class="Bool (strict)"("Visible"=w354) -> ()  [unwired: 2 in, 2 out]
            n204 = property on="Test Ring" class="Ring (strict)"("Visible"=w354) -> ()  [unwired: 2 in, 2 out]
          }
          frame "Relay", "Solenoid" {
            w357 = FALSE ("Visible")
            n205 = property on="Motor" class="Clust (strict)"("Visible"=w357) -> ()  [unwired: 2 in, 2 out]
            n206 = property on="Test Slider" class="Slide (strict)"("Visible"=w357) -> ()  [unwired: 2 in, 2 out]
            n207 = Search and Replace String(input string=w358, search string="/Value  **", replace string="/Direction") -> (result string=w364:string)  [unwired: 5 in, 3 out]
            n208 = property on="Test Ring" class="Ring (strict)"("Visible"=w357) -> ()  [unwired: 2 in, 2 out]
            n209 = call <vilib>:"NT Read String.vi"("Name"=w364) -> ("String"=w362:string)  [unwired: 9 in, 1 out]
            n210 = Equal?(x="Both directions", y=w362) -> (x = y?=w360:bool)
            n211 = Not(x=w360) -> (.not. x?=w361:bool)
            n212 = property on="Rev/Fwd" class="Clust (strict)"("Visible"=w360) -> ()  [unwired: 2 in, 2 out]
            n213 = property on="On/Off" class="Bool (strict)"("Visible"=w361, "Caption.Text"=w359) -> ()  [unwired: 2 in, 2 out]
          }
          frame "Compressor", "Digital Out" {
            w367 = FALSE ("Visible")
            # "Get direction and finish"
            n214 = property on="Motor" class="Clust (strict)"("Visible"=w367) -> ()  [unwired: 2 in, 2 out]
            n215 = property on="Test Slider" class="Slide (strict)"("Visible"=w367) -> ()  [unwired: 2 in, 2 out]
            n216 = property on="Test Ring" class="Ring (strict)"("Visible"=w367) -> ()  [unwired: 2 in, 2 out]
            n217 = property on="On/Off" class="Bool (strict)"("Visible"=TRUE, "Caption.Text"=w368) -> ()  [unwired: 2 in, 2 out]
            n218 = property on="Rev/Fwd" class="Clust (strict)"("Visible"=FALSE) -> ()  [unwired: 2 in, 2 out]
          }
          frame "Camera" {
            n219 = call <vilib>:"Get Last Path Segment.vi"("String in"=w375) -> ("String out"=w376:string)  [unwired: 10 in]
            n220 = property on="On/Off" class="Bool (strict)"("Visible"=FALSE) -> ()  [unwired: 2 in, 2 out]
            n221 = property on="Motor" class="Clust (strict)"("Visible"=FALSE) -> ()  [unwired: 2 in, 2 out]
            n222 = property on="Rev/Fwd" class="Clust (strict)"("Visible"=FALSE) -> ()  [unwired: 2 in, 2 out]
            n223 = case shown="\"White Balance  **\"" w376 {
              tunnel: w375 -> [w382 w391 w400 w409 w418 _ w424]
              tunnel: w374 -> [w380 w388 w397 w406 w415 _ _]
              frame "Size  **" {
                n224 = Index Array(array=w380) -> (element=w379:cluster{string[]})  [unwired: 1 in]
                n225 = call <vilib>:"NT Read String.vi"("Name"=w382) -> ("String"=w381:string)  [unwired: 9 in, 1 out]
                n226 = Unbundle(w379) -> (w377:string[])
                n227 = Match First String(2:w377, 3:w381) -> (0:w378:i32)  [unwired: 1 out]
                n228 = property on="Test Ring" class="Ring (strict)"("Value"=w378, "Strings []"=w377) -> ()  [unwired: 2 in, 2 out]
                n229 = property on="Test Ring" class="Ring (strict)"("Visible"=TRUE) -> ()  [unwired: 2 in, 2 out]
                n230 = property on="Test Slider" class="Slide (strict)"("Visible"=FALSE) -> ()  [unwired: 2 in, 2 out]
              }
              frame "White Balance  **" {
                n231 = Index Array(array=w388, index=1) -> (element=w389:cluster{string[]})
                n232 = call <vilib>:"NT Read String.vi"("Name"=w391) -> ("String"=w390:string)  [unwired: 9 in, 1 out]
                n233 = Unbundle(w389) -> (w386:string[])
                n234 = Match First String(2:w386, 3:w390) -> (0:w385:i32)  [unwired: 1 out]
                n235 = property on="Test Ring" class="Ring (strict)"("Value"=w385, "Strings []"=w386) -> ()  [unwired: 2 in, 2 out]
                n236 = property on="Test Ring" class="Ring (strict)"("Visible"=TRUE) -> ()  [unwired: 2 in, 2 out]
                n237 = property on="Test Slider" class="Slide (strict)"("Visible"=FALSE) -> ()  [unwired: 2 in, 2 out]
              }
              frame "Exposure  **" {
                n238 = Index Array(array=w397, index=2) -> (element=w398:cluster{string[]})
                n239 = call <vilib>:"NT Read String.vi"("Name"=w400) -> ("String"=w399:string)  [unwired: 9 in, 1 out]
                n240 = Unbundle(w398) -> (w394:string[])
                n241 = Match First String(2:w394, 3:w399) -> (0:w395:i32)  [unwired: 1 out]
                n242 = property on="Test Ring" class="Ring (strict)"("Value"=w395, "Strings []"=w394) -> ()  [unwired: 2 in, 2 out]
                n243 = property on="Test Ring" class="Ring (strict)"("Visible"=TRUE) -> ()  [unwired: 2 in, 2 out]
                n244 = property on="Test Slider" class="Slide (strict)"("Visible"=FALSE) -> ()  [unwired: 2 in, 2 out]
              }
              frame "Exposure Priority  **" {
                n245 = Index Array(array=w406, index=3) -> (element=w407:cluster{string[]})
                n246 = call <vilib>:"NT Read String.vi"("Name"=w409) -> ("String"=w408:string)  [unwired: 9 in, 1 out]
                n247 = Unbundle(w407) -> (w403:string[])
                n248 = Match First String(2:w403, 3:w408) -> (0:w404:i32)  [unwired: 1 out]
                n249 = property on="Test Ring" class="Ring (strict)"("Value"=w404, "Strings []"=w403) -> ()  [unwired: 2 in, 2 out]
                n250 = property on="Test Ring" class="Ring (strict)"("Visible"=TRUE) -> ()  [unwired: 2 in, 2 out]
                n251 = property on="Test Slider" class="Slide (strict)"("Visible"=FALSE) -> ()  [unwired: 2 in, 2 out]
              }
              frame "Color Enable  **" {
                n252 = Index Array(array=w415, index=4) -> (element=w416:cluster{string[]})
                n253 = call <vilib>:"NT Read String.vi"("Name"=w418) -> ("String"=w417:string)  [unwired: 9 in, 1 out]
                n254 = Unbundle(w416) -> (w412:string[])
                n255 = Match First String(2:w412, 3:w417) -> (0:w413:i32)  [unwired: 1 out]
                n256 = property on="Test Ring" class="Ring (strict)"("Value"=w413, "Strings []"=w412) -> ()  [unwired: 2 in, 2 out]
                n257 = property on="Test Ring" class="Ring (strict)"("Visible"=TRUE) -> ()  [unwired: 2 in, 2 out]
                n258 = property on="Test Slider" class="Slide (strict)"("Visible"=FALSE) -> ()  [unwired: 2 in, 2 out]
              }
              frame Default {
                n259 = property on="Test Ring" class="Ring (strict)"("Visible"=FALSE) -> ()  [unwired: 2 in, 2 out]
                n260 = property on="Test Slider" class="Slide (strict)"("Visible"=FALSE) -> ()  [unwired: 2 in, 2 out]
              }
              frame "Brightness  **", "Color Level  **", "Compression  **", "FPS  **", "Sharpness  **" {
                n261 = call <vilib>:"NT Read Number.vi"("Name"=w424) -> ("Numeric"=w423:dbl)  [unwired: 9 in, 1 out]
                n262 = local write "Test Slider"(w423) -> ()
                n263 = property on="Test Slider" class="Slide (strict)"("Visible"=TRUE, "Scale.Maximum"=100.0 ("Scale.Range:Maximum")) -> ()  [unwired: 2 in, 2 out]
                n264 = property on="Test Ring" class="Ring (strict)"("Visible"=FALSE) -> ()  [unwired: 2 in, 2 out]
              }
            }
          }
        }
        n265 = property on="Progress" class="Clust (strict)"("Visible"=FALSE) -> ()  [unwired: 2 in, 2 out]
      }
      event "Test Name": Mouse Enter {
        # "Populate the ring with the list of tests"
        n266 = event-data() -> ()  [unwired: 1 in, 1 out]
        n267 = call <vilib>:"NT Read String Array.vi"("Name"="TestMode/TestList") -> ("String Array"=w432:string[])  [unwired: 9 in, 1 out]
        n268 = Build Array (concatenate)("Select the test to run...", w432) -> (w431:string[])
        n269 = property on="Test Name" class="Ring (strict)"("Strings []"=w431) -> ()  [unwired: 2 in, 2 out]
      }
      event "Test Name": Value Change {
        w434 = FALSE ("Visible")
        # "Tell the robot the test name to run"
        n270 = event-data() -> ("NewVal"=w438:u16)  [unwired: 1 in]
        n271 = property on="Test Name" class="Ring (strict)"() -> ("Strings []"=w439:string[])  [unwired: 2 in, 2 out]
        n272 = local write "Progress"(T6 {"Test Progress"=0, "Test Progress Text"=""} ("Progress")) -> ()
        n273 = Index Array(array=w439, index=w438) -> (element=w437:string)
        n274 = call <vilib>:"NT Write String.vi"("String"=w437, "Name"="TestMode/TestName") -> ()  [unwired: 9 in, 1 out]
        n275 = property on="Progress" class="Clust (strict)"("Visible"=TRUE) -> ()  [unwired: 2 in, 2 out]
        n276 = property on="Motor" class="Clust (strict)"("Visible"=w434) -> ()  [unwired: 2 in, 2 out]
        n277 = property on="Test Slider" class="Slide (strict)"("Visible"=w434) -> ()  [unwired: 2 in, 2 out]
        n278 = property on="On/Off" class="Bool (strict)"("Visible"=w434) -> ()  [unwired: 2 in, 2 out]
        n279 = property on="Rev/Fwd" class="Clust (strict)"("Visible"=w434) -> ()  [unwired: 2 in, 2 out]
        n280 = property on="Test Ring" class="Ring (strict)"("Visible"=w434) -> ()  [unwired: 2 in, 2 out]
      }
      event "Select Auto": Mouse Enter {
        # "Populate the combo box with the list of autonomous options"
        n281 = event-data() -> ()  [unwired: 1 in, 1 out]
        n282 = call <vilib>:"NT Read String Array.vi"("Name"="Auto List") -> ("String Array"=w441:string[])  [unwired: 9 in, 1 out]
        n283 = property on="Select Auto" class="CmbBox"("Strings[]"=w441) -> ()  [unwired: 2 in, 2 out]
      }
      event "Select Auto": Value Change {
        # "User modified the Auto Selection. Write to NT variable so robot knows."
        n284 = event-data() -> ("NewVal"=w444:string)  [unwired: 1 in]
        n285 = call <vilib>:"NT Write String.vi"("String"=w444, "Name"="Auto Selector") -> ()  [unwired: 9 in, 1 out]
      }
      event "Command Selection": Value Change {
        # "Get the params and show in table"
        n286 = event-data() -> ("NewVal"=w450:i32)  [unwired: 1 in]
        n287 = property on="Command Selection" class="MCListbox (strict)"() -> ("ItemNames"=w448:string[][])  [unwired: 2 in, 2 out]
        n288 = call <vilib>:"WPI_DashboardUpdate Command Params.vi"("NewVal"=w450, "Commands"=w448, "Param Tbl"=w449) -> ()  [unwired: 8 in, 1 out]
      }
      event "Execute Command": Value Change {
        # "Started one, Unique ID holds\nresponse"
        n289 = event-data() -> ()  [unwired: 1 in, 1 out]
        n290 = property on="Command Selection" class="MCListbox (strict)"() -> ("ItemNames"=w461:string[][])  [unwired: 2 in, 2 out]
        n291 = Index Array(array=w461, index (row)="Command Selection", index (col)=0) -> (element=w459:string)
        n292 = call <vilib>:"Invoke Commands.vi"("Command Params"="Command Params", "Function Name"=w459) -> ("Params"=w455:u8, "Started"=w454:bool)  [unwired: 7 in, 1 out]
        n293 = Array Subset(array="Command Params", length (row)=w455) -> (w456:string[][])  [unwired: 3 in]
        n294 = Select(t="Executing" ("Cmd Status"), s=w454, f="" ("Cmd Status")) -> (s? t:f=→"Cmd Status":string)
      }
      event "Command Selection": Double Click {
        n295 = event-data() -> ("Row"=w469:i32)  [unwired: 1 in]
        n296 = property on="Command Selection" class="MCListbox (strict)"() -> ("ItemNames"=w472:string[][])  [unwired: 2 in, 2 out]
        n297 = local read "Command Params"() -> (w468:string[][])
        n298 = Index Array(array=w472, index (row)=w469, index (col)=0) -> (element=w470:string)
        n299 = call <vilib>:"Invoke Commands.vi"("Command Params"=w468, "Function Name"=w470) -> ("Params"=w467:u8, "Started"=w462:bool)  [unwired: 7 in, 1 out]
        n300 = Array Subset(array=w468, length (row)=w467) -> (w466:string[][])  [unwired: 3 in]
        n301 = Select(t="Executing" ("Cmd Status"), s=w462, f="" ("Cmd Status")) -> (s? t:f=w463:string)
        n302 = local write "Cmd Status"(w463) -> ()
      }
      event "CheckList": Double Click {
        # "Shift clears all"
        # "Update symbols on the listbox"
        n303 = event-data() -> ("PlatMods.Shift"=w474:bool, "Row"=w476:i32)  [unwired: 1 in]
        n304 = case shown="True" w474 {
          tunnel: w476 -> [w480 _]
          tunnel: 1 -> [w479 _]
          frame False {
            n305 = property on="CheckList" class="LstBox (strict)"() -> ("Item Symbols"=w478:i32[])  [unwired: 2 in, 2 out]
            n306 = Replace Array Subset(array=w478, new element=w479, index=w480) -> (w477:i32[])
            n307 = property on="CheckList" class="LstBox (strict)"("Item Symbols"=w477) -> ()  [unwired: 2 in, 2 out]
          }
          frame True {
            w481 = 0 ("Top Row")
            n308 = property on="CheckList" class="LstBox (strict)"() -> ("Number of Rows"=w483:u32)  [unwired: 2 in, 2 out]
            n309 = Initialize Array(0, w483) -> (w482:i32[])
            n310 = property on="CheckList" class="LstBox (strict)"("Top Row"=w481, "Value"=w481, "Item Symbols"=w482) -> ()  [unwired: 2 in, 2 out]
          }
        }
      }
      event "CheckList": Key Down {
        # "Update symbols on the listbox\nLeft and right keys check and uncheck"
        n311 = event-data() -> ("VKey"=w487:T23)  [unwired: 1 in]
        n312 = case shown="\"Left\", \"Right\"" w487 {
          selector: w487 -> [w492 _]
          tunnel: eventvkey."Left" ("VKey") -> [w490 _]
          frame "Left", "Right" {
            n313 = Equal?(x=w490, y=w492) -> (x = y?=w491:bool)
            n314 = Select(t=0, s=w491, f=1) -> (s? t:f=w493:i32)
            n315 = property on="CheckList" class="LstBox (strict)"() -> ("Item Symbols"=w496:i32[])  [unwired: 2 in, 2 out]
            n316 = Replace Array Subset(array=w496, new element=w493, index="CheckList") -> (w495:i32[])
            n317 = property on="CheckList" class="LstBox (strict)"("Item Symbols"=w495) -> ()  [unwired: 2 in, 2 out]
          }
          frame Default {
          }
        }
      }
      event "Motor.Enable": Value Change {
        # "When the test mode otor enable helper is set, update that\ntree row item's value"
        n318 = event-data() -> ("NewVal"=w502:bool)  [unwired: 1 in]
        n319 = Unbundle("Motor") -> ("Value"=w501:dbl)  [unwired: 1 out]
        n320 = Select(t=w501, s=w502, f=0.0) -> (s? t:f=w499:dbl)
        n321 = call <vilib>:"NT Write Number.vi"("Numeric"=w499, "Name"=w498) -> ()  [unwired: 9 in, 1 out]
      }
      event "Test Slider": Value Change {
        # "When the test mode slider helper is set, update that\ntree row item's value"
        n322 = event-data() -> ("NewVal"=w505:dbl)  [unwired: 1 in]
        n323 = call <vilib>:"NT Write Number.vi"("Numeric"=w505, "Name"=w506) -> ()  [unwired: 9 in, 1 out]
      }
      event "On/Off": Value Change {
        # "When the test mode on/off helper value is set, update that\ntree row item's value"
        n324 = event-data() -> ("NewVal"=w510:bool)  [unwired: 1 in]
        n325 = Boolean To (0,1)(Boolean=w510) -> (0, 1=w509:i16)
        n326 = call <vilib>:"NT Write Number.vi"("Numeric"=w509, "Name"=w508) -> ()  [unwired: 9 in, 1 out]
      }
      event "Rev/Fwd": Value Change {
        # "When the test mode helper value for relays is set, update that\ntree row item's value"
        n327 = event-data() -> ("NewVal.Forward"=w518:bool, "NewVal.Reverse"=w517:bool)  [unwired: 1 in]
        n328 = Boolean To (0,1)(Boolean=w518) -> (0, 1=w514:i16)
        n329 = Boolean To (0,1)(Boolean=w517) -> (0, 1=w516:i16)
        n330 = Negate(x=w516) -> (-x=w515:i16)
        n331 = Add(x=w514, y=w515) -> (x+y=w513:i16)
        n332 = call <vilib>:"NT Write Number.vi"("Numeric"=w513, "Name"=w512) -> ()  [unwired: 9 in, 1 out]
      }
      event "Test Ring": Value Change {
        # "When a test mode helper value is selected from the ring,\nset the tree item's variable to the string value"
        n333 = event-data() -> ("NewVal"=w522:u16)  [unwired: 1 in]
        n334 = property on="Test Ring" class="Ring (strict)"() -> ("Strings []"=w523:string[])  [unwired: 2 in, 2 out]
        n335 = Index Array(array=w523, index=w522) -> (element=w521:string)
        n336 = call <vilib>:"NT Write String.vi"("String"=w521, "Name"=w520) -> ()  [unwired: 9 in, 1 out]
      }
      event "Rec Mode": Value Change {
        # "Update globals for recording mode and path to read log from.\nClear when logging and let NetworkTables set path for vision to\nuse."
        n337 = event-data() -> ("NewVal"=w534:enum32{"Stop", "Record", "Playback"})  [unwired: 1 in]
        n338 = global write "WPI_DashboardLogging Global.vi" "Logging Filename"(path "") -> ()
        n339 = global write "WPI_DashboardLogging Global.vi" "Recording"(w534) -> ()
        n340 = case shown="\"Playback\"" w534 {
          tunnel: w533 -> [_ w536 w545]
          tunnel: [_ _ w544] -> w531
          tunnel: [_ _ w543] -> _
          tunnel: w529 -> [_ _ w541]
          tunnel: cluster{i32, i32} {-250, 170} -> [_ _ w540]
          tunnel: [_ _ T24 {"Image Size"=TRUE, "Image Type"=TRUE, "Pixel Value"=TRUE, "ROI Information"=TRUE, "Zoom Factor"=FALSE} ("Image Information Shown:All Elements")] -> w524
          tunnel: [_ _ TRUE ("Zoom Factor")] -> w525
          tunnel: w527 -> [_ _ w537]
          frame Default {
          }
          frame "Stop", "Record" {
            # "Place Window too"
            n341 = invoke class="VI" method="FP.Close"(reference=w536) -> (reference out=w535:refnum<vi>)  [unwired: 2 in, 2 out]
            n342 = invoke class="VI" method="Abort VI"(reference=w535) -> ()  [unwired: 2 in, 3 out]
          }
          frame "Playback" {
            n343 = call "Open Playback Panel.vi"("Offset"=w540, "DB VI Ref"=w541, "Playback in"=w545) -> ("Playback out"=w542:refnum<vi>)  [unwired: 8 in]
            n344 = register-events(w542, w537) -> (reference out=w544:refnum<event-registration>, error out=w543:errorcluster)  [unwired: 2 in]
          }
        }
        n345 = property on="Camera Image Right" class="ImageControl"("Image Information Shown"=w524, "Image Information Visible"=w525) -> ()  [unwired: 2 in, 2 out]
        n346 = property on="Camera Image" class="ImageControl"("Image Information Shown"=w524, "Image Information Visible"=w525) -> ()  [unwired: 2 in, 2 out]
        n347 = call <vilib>:"WPI_DashboardNT Log FieldName Cache.vi"("Operation"=enum16{"Lookup/Add", "Index", "Clear"}."Clear") -> ()  [unwired: 8 in, 3 out]
      }
      event Panel Close {
        w547 = enum32{"Stop", "Record", "Playback"}."Stop" ("Rec Mode")
        # "Playback window has been closed, abort"
        n348 = event-data() -> ()  [unwired: 1 in, 4 out]
        n349 = local write "Rec Mode"(w547) -> ()
        n350 = global write "WPI_DashboardLogging Global.vi" "Recording"(w547) -> ()
      }
      event Panel Close {
        # "Abort playback window and ourself"
        n351 = event-data() -> ()  [unwired: 1 in, 4 out]
        n352 = invoke class="VI" method="FP.Close"(reference=w551) -> (reference out=w550:refnum<vi>)  [unwired: 2 in, 2 out]
        n353 = invoke class="VI" method="Abort VI"(reference=w550) -> (error out=w549:errorcluster)  [unwired: 2 in, 2 out]
        n354 = invoke class="VI" method="Abort VI"(error in=w549) -> ()  [unwired: 2 in, 3 out]
      }
      event User Event {
        n355 = event-data() -> ("IDs"=w558:cluster{"RPC field ID":u16, "Unique ID":u16}, "String"=w557:string)  [unwired: 1 in]
        n356 = Bundle("IDs"=w558, "String"=w557) -> (w556:T10)  [unwired: 1 in]
        n357 = call <vilib>:"Retrieve RPC Response.vi"("RPC Response"=w556) -> ("Output"=w554:string[][])  [unwired: 10 in]
        n358 = Build Array (concatenate)(w552, w554) -> (w553:string[][])
        n359 = local write "Command Params"(w553) -> ()
        n360 = local write "Cmd Status"("" ("Cmd Status")) -> ()
      }
      event "Tree": Double Click {
        n361 = event-data() -> ("PlatMods"=w564:T27, "Tag"=w561:string)  [unwired: 1 in]
        n362 = Unbundle(w564) -> ("Shift"=w563:bool)  [unwired: 4 out]
        n363 = String Subset(string=w561, length (rest)=1 ("length (rest)")) -> (substring=w560:string)  [unwired: 1 in]
        n364 = Not(x=w563) -> (.not. x?=w562:bool)
        n365 = case shown="\"/\"" w560 {
          tunnel: w561 -> [_ w567]
          tunnel: w562 -> [_ w566]
          frame Default {
          }
          frame "/" {
            n366 = call <vilib>:"NT Update Persistence.vi"("Persistence"=w566, "Name"=w567) -> ()  [unwired: 9 in, 1 out]
          }
        }
      }
    }
  }
  n367 = while {
    tunnel: w65 -> [w569]
    i -> [w572]
    stop <- FALSE stop-if-true
    n368 = Wait (ms)(milliseconds to wait=u32 100) -> ()  [unwired: 1 out]
    n369 = case shown="\"Playback\"" "Rec Mode" {
      tunnel: w572 -> [_ _ w587]
      tunnel: [u32 2829099 ("Base Color") u32 11141120 ("Target Color") w576] -> w568
      frame "Stop", Default {
        # "Reset the color, extra updates don't cost much"
      }
      frame "Record" {
      }
      frame "Playback" {
        # "Playback"
        n370 = Quotient & Remainder(x=w587, y=u32 50 ("milliseconds to wait")) -> (x-y*floor(x/y)=w583:u32)  [unwired: 1 out]
        n371 = Divide(x=w583, y=u32 50 ("milliseconds to wait")) -> (x/y=w580:dbl)
        n372 = Multiply(x=6.283185307179586, y=w580) -> (x*y=w585:dbl)
        n373 = Sine(x=w585) -> (sin(x)=w584:dbl)
        n374 = Absolute Value(x=w584) -> (abs(x)=w577:dbl)
        n375 = call "Interpolate RGB Color.vi"("Proportion"=w577, "Target Color"=u32 30976, "Base Color"=u32 2829099) -> ("Result Color"=w576:u32)  [unwired: 8 in]
      }
    }
    n376 = property class="Pane"(reference=w569, "PaneColor"=w568) -> ()  [unwired: 1 in, 2 out]
  }
  n377 = local write "Dashboard Tab"(T8."Drive" ("Dashboard Tab")) -> ()
  n378 = property on="On/Off" class="Bool (strict)"("Visible"=w36) -> ()  [unwired: 2 in, 2 out]
  n379 = property on="Motor" class="Clust (strict)"("Visible"=w36) -> ()  [unwired: 2 in, 2 out]
  n380 = property on="Progress" class="Clust (strict)"("Visible"=w36) -> ()  [unwired: 2 in, 2 out]
  n381 = property on="Test Ring" class="Ring (strict)"("Visible"=w36) -> ()  [unwired: 2 in, 2 out]
  n382 = property on="Rev/Fwd" class="Clust (strict)"("Visible"=w36) -> ()  [unwired: 2 in, 2 out]
  n383 = while {
    tunnel: u16 1741 ("timeout ms (25000)") -> [w589]
    stop <- FALSE stop-if-true
    n384 = TCP Create Listener(10:w589) -> (0:w588:errorcluster, 3:w590:refnum<k5>)  [unwired: 4 in, 1 out]
    n385 = case shown="No Error" w588 {
      selector: w588 -> [w592 _]
      tunnel: w590 -> [w593 _]
      frame No Error {
        n386 = while {
          tunnel: w593 -> [w596]
          tunnel: w592 -> [w595]
          stop <- FALSE stop-if-true
          n387 = TCP Wait On Listener(8:w595, 11:w596) -> (0:w597:errorcluster, 4:w598:refnum<k5>)  [unwired: 2 in, 3 out]
          n388 = local write "TCP"(w598) -> ()
          n389 = case shown="No Error" w597 {
            frame No Error {
            }
            frame Error {
              n390 = Wait (ms)(milliseconds to wait=u32 1000) -> ()  [unwired: 1 out]
            }
          }
        }
      }
      frame Error {
        n391 = Wait (ms)(milliseconds to wait=u32 1000) -> ()  [unwired: 1 out]
      }
    }
  }
  n392 = local write "Command Selection"(u16 0 ("milliseconds to wait")) -> ()
  n393 = local write "Command Params"(string[][] [] ("Command Params")) -> ()
  n394 = global write "WPI_DashboardLogging Global.vi" "Recording"(w59) -> ()
  n395 = local write "Rec Mode"(w59) -> ()
  n396 = call <vilib>:"NT Write String.vi"("String"="Select Auto", "Name"="Auto Selector") -> ()  [unwired: 9 in, 1 out]
